vi "UIRef.vi"(8 "error in":errorcluster, 11 "fixed channel editor in":refnum<class "My Awesome Control Modules editor node.lvclass">) -> (0 "error out":errorcluster, 2 "VI refnum":refnum<vi>, 3 "fixed channel editor out":refnum<class "My Awesome Control Modules editor node.lvclass">)   [LabVIEW 2013, in "My Awesome Control Modules editor node.lvclass"]
uses:
  My Awesome Control Modules editor node.lvclass
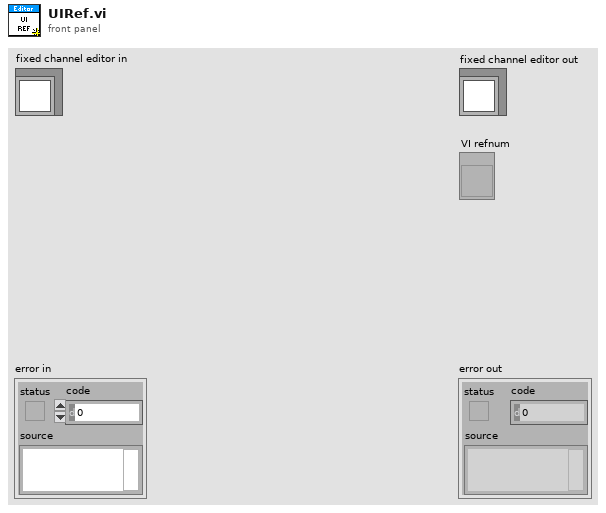
[diagram p1: front panel]
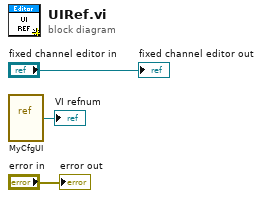
[diagram p0: block diagram]
diagram:
  n1 = vi-ref "MyCfgUI.vi"() -> (→"VI refnum":refnum<vi>)
  "error out" <- "error in"
  "fixed channel editor out" <- "fixed channel editor in"
